vi "Parse Subsystem Name.vi"(1 "Action Enum":T1=enum."Drive Left") -> (0 "Subsystem Name":string)   [LabVIEW 2015, in "Sprocket.lvlib"]
uses:
  lib/Sprocket.lvlib
  Action/Action Name.ctl
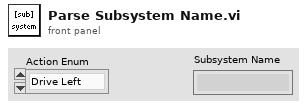
[diagram p1: front panel]
types:
  T1 = typedef "Sprocket.lvlib/Action Name.ctl" = enum16{"No Action", "Drive Left", "Drive Right"}
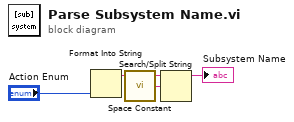
[diagram p0: block diagram]
diagram:
  n1 = Format Into String("Action Enum") -> (resulting string=w3:string)  [unwired: 3 in, 1 out]
  n2 = call <vilib>:"Space Constant.vi"() -> ("String"=w2:string)
  n3 = Search/Split String(string=w3, search string/char (-)=w2) -> (substring before match=→"Subsystem Name":string)  [unwired: 1 in, 2 out]
